vi "Binary Actor.vi"(11 "VISA resource name":refnum<visa-resource-name>) -> (0 "error out":errorcluster)   [LabVIEW 2019, in "Binary Actor.lvlib"]
uses:
  Binary Actor.lvlib
  Queue Task.ctl
  Actor Command.ctl
  Actor Task.ctl
  <vilib>/Instr/_visa.llb/VISA Configure Serial Port (Instr).vi
  <vilib>/Utility/miscctls.llb/LVMapReplaceAction.ctl
panel:
  out "read buffer":string
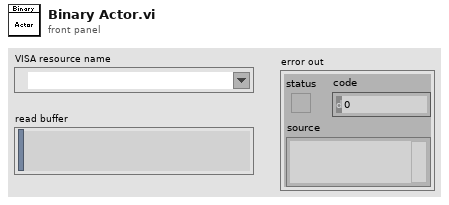
[diagram p1: front panel]
types:
  T1 = typedef "Binary Actor.lvlib/Actor Command.ctl" = cluster{"Task":T2, "Data":string, "Response Queue":refnum<queue>}
  T2 = typedef "Binary Actor.lvlib/Actor Task.ctl" = enum8{"Write", "Get Data", "Stop"}
  T3 = typedef "Binary Actor.lvlib/Queue Task.ctl" = enum8{"Get Reference", "Send", "Close"}
  T4 = typedef "LVMapReplaceAction.ctl" = enum32{"Modify Entry only if found", "Add or Modify Entry", "Delete Entry"}
  T5 = typedef "ASCII Actor.lvlib/Actor Command.ctl" = cluster{"Task":T6, "Data":string, "Response Queue":refnum<queue>}
  T6 = typedef "ASCII Actor.lvlib/Actor Task.ctl" = enum8{"Write", "Get Data", "Stop"}
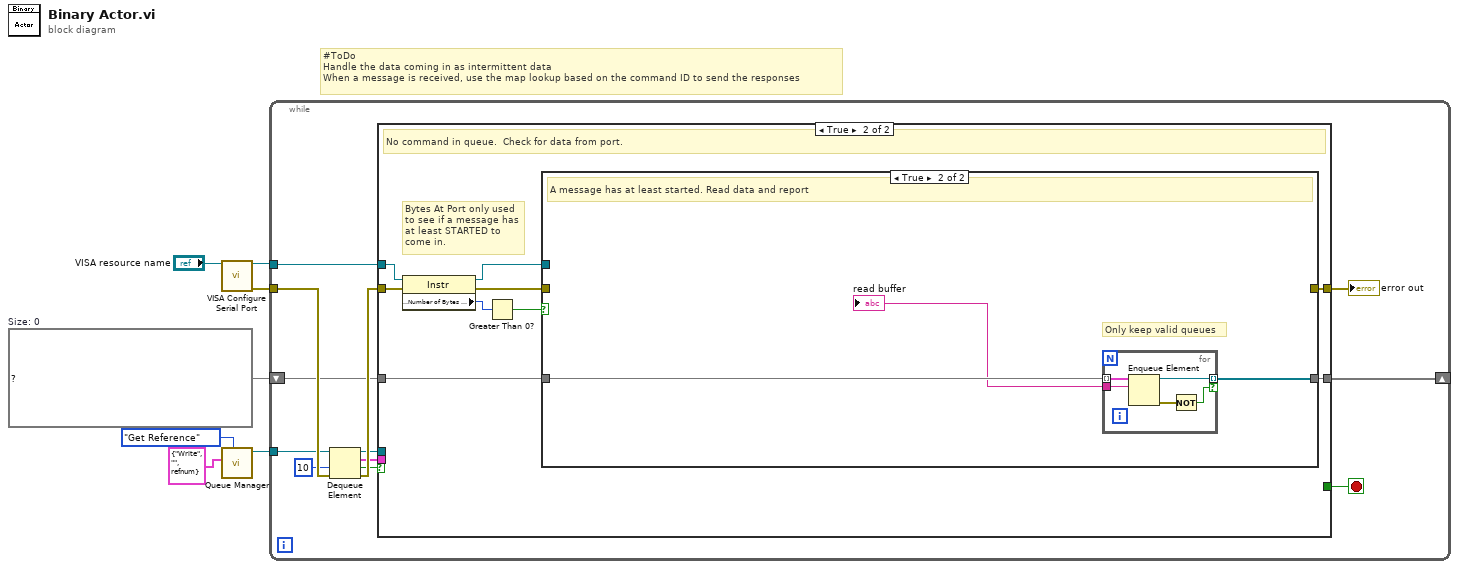
[diagram p0: block diagram]
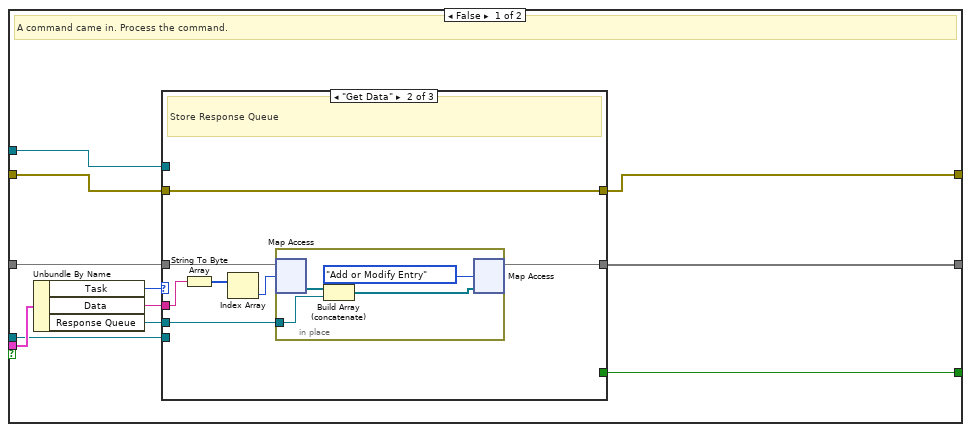
[diagram p2: hidden frame]
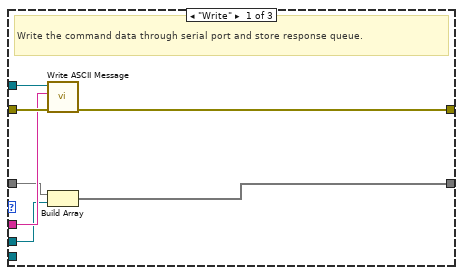
[diagram p3: hidden frame]
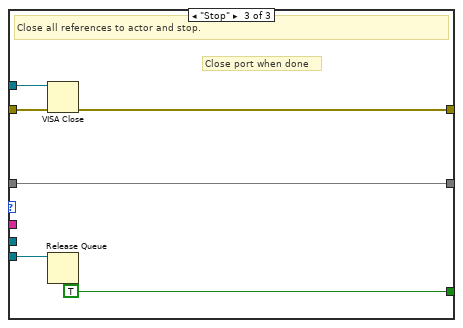
[diagram p4: hidden frame]
diagram:
  w1 = map{u8, refnum<queue>[]} {}  # Size: 0
  # "#ToDo\nHandle the data coming in as intermittent data\nWhen a message is received, use the map lookup based on the command ID to send the responses"
  n1 = call-poly "VISA Configure Serial Port"("VISA resource name"="VISA resource name") -> ("VISA resource name out"=w5:refnum<visa-resource-name>, "error out"=w7:errorcluster)  [unwired: 13 in]
  n2 = call "Queue Manager.vi"("Task"=Queue_Task."Get Reference", "Command"=T1 {"Task"=enum."Write", "Data"="", "Response Queue"=refnum}) -> ("Queue"=w4:refnum<queue>)  [unwired: 8 in, 1 out]
  n3 = while {
    tunnel: w7 -> [w18]
    tunnel: w5 -> [w16]
    tunnel: w4 -> [w15]
    shift-right: [w10] -> _
    shift-left: w1 -> [w11]
    stop <- w8 stop-if-true
    n4 = Dequeue Element(queue=w15, timeout in ms (-1)=10, error in (no error)=w18) -> (queue out=w9:refnum<queue>, element=w12:T5, timed out?=w13:bool, error out=w19:errorcluster)
    n5 = case shown="True" w13 {
      tunnel: [w29 w62] -> w17
      tunnel: w16 -> [w24 w60]
      tunnel: w19 -> [w30 w61]
      tunnel: w12 -> [w28 _]
      tunnel: w11 -> [w23 w56]
      tunnel: [w22 w55] -> w10
      tunnel: w9 -> [w21 _]
      tunnel: [w20 _] -> w8
      frame False {
        # "A command came in. Process the command."
        n6 = Unbundle By Name(w28) -> ("Task"=w25:T6, "Data"=w26:string, "Response Queue"=w27:refnum<queue>)
        n7 = case shown="\"Get Data\"" w25 {
          tunnel: w27 -> [w32 w39 _]
          tunnel: w26 -> [w34 w42 _]
          tunnel: w24 -> [w35 _ w52]
          tunnel: w23 -> [w33 w43 w50]
          tunnel: [w31 w38 w50] -> w22
          tunnel: w30 -> [w37 w44 w54]
          tunnel: [w36 w44 w53] -> w29
          tunnel: w21 -> [_ _ w51]
          tunnel: [_ _ TRUE] -> w20
          frame "Write" {
            # "Write the command data through serial port and store response queue."
            n8 = call "Write ASCII Message.vi"("error in"=w37, "Message"=w34, "VISA resource in"=w35) -> ("error out"=w36:errorcluster)  [unwired: 7 in, 1 out]
            n9 = Build Array(w33, w32) -> (w31:map{u8, refnum<queue>[]}[])
          }
          frame "Get Data" {
            # "Store Response Queue"
            n10 = String To Byte Array(string=w42) -> (unsigned byte array=w41:u8[])
            n11 = Index Array(array=w41) -> (element=w40:u8)  [unwired: 1 in]
            n12 = in-place {
              in-place-border: w39 -> [w46]
              n13 = in-place-map #1(w43, w40) -> (w47:refnum<queue>[])  [unwired: 1 in, 1 out]
              n14 = Build Array (concatenate)(w47, w46) -> (w45:refnum<queue>[])
              n15 = in-place-map #1(w45, LVMapReplaceAction."Add or Modify Entry" ("action")) -> (w38:map{u8, refnum<queue>[]})  [unwired: 2 out]
            }
          }
          frame "Stop" {
            # "Close port when done"
            # "Close all references to actor and stop."
            n16 = VISA Close(VISA resource name=w52, error in (no error)=w54) -> (error out=w53:errorcluster)
            n17 = Release Queue(queue=w51) -> ()  [unwired: 2 in, 3 out]
          }
        }
      }
      frame True {
        # "Bytes At Port only used\nto see if a message has\nat least STARTED to\ncome in."
        # "No command in queue.  Check for data from port."
        n18 = property class="Instr"(reference=w60, error in=w61) -> (reference out=w57:refnum<visa-resource-name>, error out=w63:errorcluster, "Serial Settings:Number of Bytes at Serial Port"=w59:u32)
        n19 = Greater Than 0?(x=w59) -> (x > 0?=w58:bool)
        n20 = case shown="True" w58 {
          tunnel: w63 -> [w65 _]
          tunnel: w57 -> [_ _]
          tunnel: [w65 w69] -> w62
          tunnel: w56 -> [w64 w68]
          tunnel: [w64 w66] -> w55
          frame False {
            # "No message. Go back to waiting for a command."
          }
          frame True {
            # "Only keep valid queues"
            # "A message has at least started. Read data and report"
            n21 = for {
              tunnel: w68 -> [w73] mode=indexing
              tunnel: [w72] -> w67
              tunnel: [w71] -> w66 mode=indexing if=w70
              n22 = Enqueue Element(queue=w73, element=w72) -> (queue out=w71:refnum<queue>, error out=w74:errorcluster)  [unwired: 2 in, 1 out]
              n23 = Not(x=w74) -> (.not. x?=w70:bool)
            }
            "read buffer" <- w67
          }
        }
      }
    }
    "error out" <- w17
  }
